vi "Calculul FFT bilaterală.vi"() -> ()   [LabVIEW 2011]
uses:
  <vilib>/Analysis/2dsp.llb/Real FFT.vi
  <vilib>/Analysis/NI_AALBase.lvlib
  <vilib>/Analysis/NI_AALPro.lvlib
panel:
  out "Spectrul":cluster{i32, dbl, dbl[]}(graph)
  out "semnalul in domeniul timp":dbl[](graph)
  in  "Amplitude":dbl
  in  "no. of samples":i32
  in  "sampling frequency [Hz]":dbl
  in  "frequency [Hz]":dbl
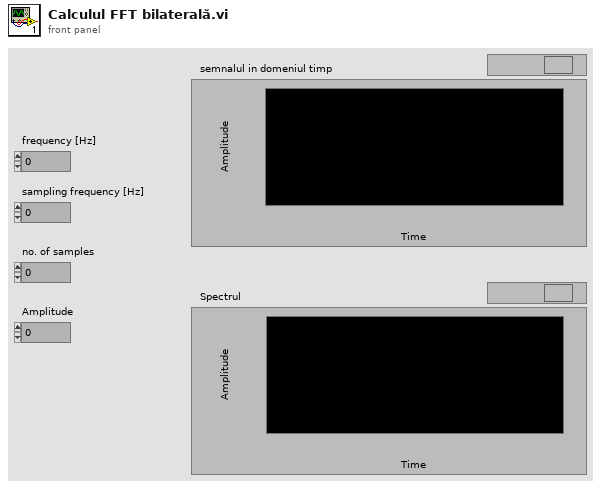
[diagram p1: front panel]
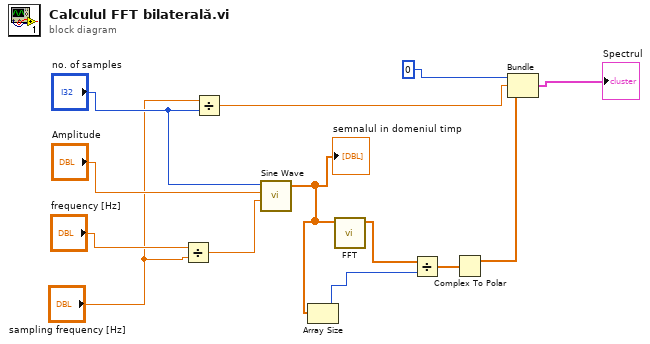
[diagram p0: block diagram]
diagram:
  n1 = Divide(x="frequency [Hz]", y="sampling frequency [Hz]") -> (x/y=w6:dbl)
  n2 = Divide(x="sampling frequency [Hz]", y="no. of samples") -> (x/y=w10:dbl)
  n3 = call <vilib>:"Sine Wave.vi"("samples"="no. of samples", "amplitude"="Amplitude", "frequency"=w6) -> ("sine wave"=w1:dbl[])  [unwired: 2 in, 2 out]
  "semnalul in domeniul timp" <- w1
  n4 = Array Size(array=w1) -> (size(s)=w8:i32)
  n5 = call-poly <vilib>:"FFT.vi"("X"=w1) -> ("FFT {X}"=w7:cdb[])  [unwired: 9 in, 1 out]
  n6 = Divide(x=w7, y=w8) -> (x/y=w13:cdb[])
  n7 = Complex To Polar(r * e^(i*theta)=w13) -> (r=w9:dbl[])  [unwired: 1 out]
  n8 = Bundle(0, w10, w9) -> (→"Spectrul":cluster{i32, dbl, dbl[]})  [unwired: 1 in]
